vi "Merge.vi"(8 "error in":errorcluster, 10 "Test Results 2":refnum<class "Test Results Base Class.lvclass">, 11 "Test Results 1":refnum<class "Test Results Base Class.lvclass">) -> (0 "error out":errorcluster, 3 "Merged\nTest Results":refnum<class "Test Results Base Class.lvclass">)   [LabVIEW 2020, in "Test Results Base Class.lvclass"]
doc: "Merge two Test Results. This VI works like \"Merge Error.vi.\" It returns the first class with a failure."
uses:
  Test Results Base Class.lvclass
  Test Results Base Class.lvclass/Test Results Base Class.ctl
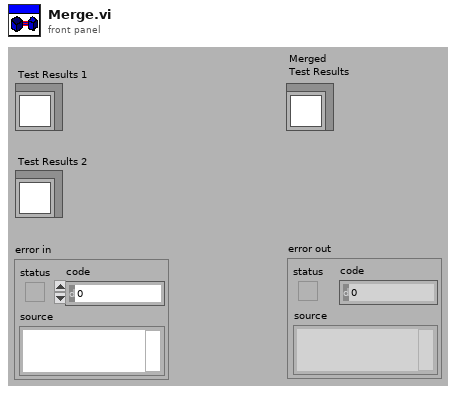
[diagram p1: front panel]
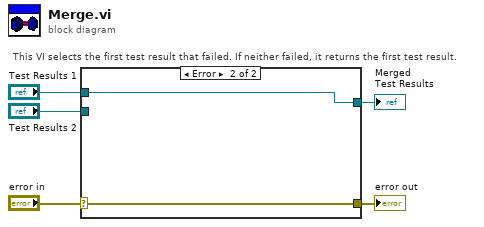
[diagram p0: block diagram]
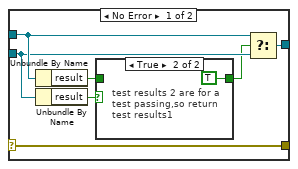
[diagram p2: hidden frame]
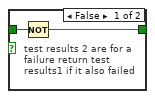
[diagram p3: hidden frame]
diagram:
  # "This VI selects the first test result that failed. If neither failed, it returns the first test result."
  n1 = case shown="Error" "error in" {
    selector: "error in" -> [w6 w17]
    tunnel: [w6 w17] -> w4
    tunnel: "Test Results 1" -> [w10 w16]
    tunnel: "Test Results 2" -> [w9 _]
    tunnel: [w11 w16] -> w1
    frame No Error {
      n2 = Unbundle By Name(w10) -> ("result"=w7:bool)
      n3 = Unbundle By Name(w9) -> ("result"=w12:bool)
      n4 = case shown="True" w12 {
        tunnel: [w13 TRUE] -> w8
        tunnel: w7 -> [w14 _]
        frame False {
          # "test results 2 are for a failure return test results1 if it also failed"
          n5 = Not(x=w14) -> (.not. x?=w13:bool)
        }
        frame True {
          # "test results 2 are for a test passing,so return test results1"
        }
      }
      n6 = Select(t=w10, s=w8, f=w9) -> (s? t:f=w11:refnum<class "Test Results Base Class.lvclass">)
    }
    frame Error {
    }
  }
  "error out" <- w4
  "Merged\nTest Results" <- w1
